vi "ErrorDialog.vi"(8 "error in":errorcluster) -> (0 "error out":errorcluster)   [LabVIEW 2010]
panel:
  out "Message":string
  in  "OK":bool
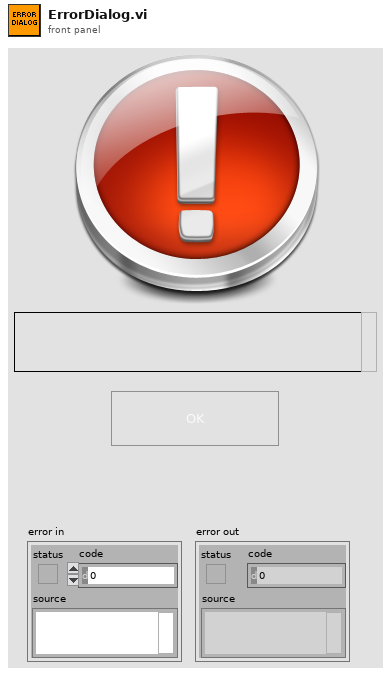
[diagram p1: front panel]
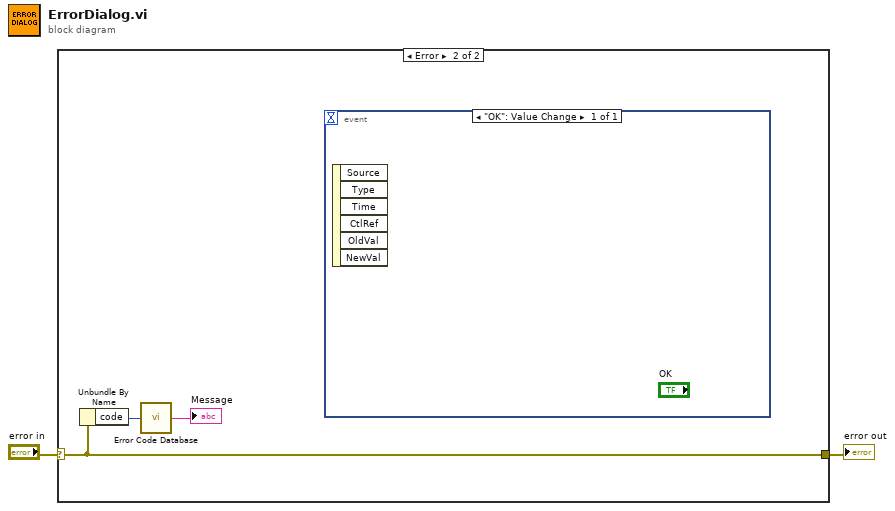
[diagram p0: block diagram]
diagram:
  n1 = case shown="Error" "error in" {
    selector: "error in" -> [w3 w6]
    tunnel: [w3 w6] -> w1
    frame No Error {
    }
    frame Error {
      n2 = Unbundle By Name(w6) -> ("code"=w5:i32)
      n3 = call <vilib>:"Error Code Database.vi"("Error Code"=w5) -> ("Error Text"=→"Message":string)
      n4 = event shown="[0] \"OK\": Value Change" {
        selector: _ -> [_]
        dyn-events: _ -> [_]
        timeout: _ -> [_]
        event "OK": Value Change {
          n5 = event-data() -> ()  [unwired: 7 out]
        }
      }
    }
  }
  "error out" <- w1
